vi "ClimberSetpointControl.vi"(11 "Buttons":bool[](array[boolean])) -> ()   [LabVIEW 2015]
uses:
  <vilib>/Rock Robotics/WPI/CAN/TalonSRX/WPI_CANTalonSRX_APIControlMode.ctl
  Utilities/MotorPositionGlobals.vi
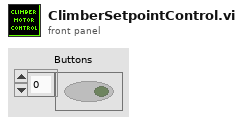
[diagram p1: front panel]
types:
  T1 = typedef "WPI_ServoDeviceRef.ctl" = cluster{"DeviceStatus":errorcluster, "PWM Channel":T2, "DeadBand":T3}
  T2 = typedef "FPGA_DIOPWMChannel.ctl" = enum8{"PWM 0", "PWM 1", "PWM 2", "PWM 3", "PWM 4", "PWM 5", "PWM 6", "PWM 7", "PWM 8", "PWM 9", "PWM MXP 0", "PWM MXP 1", "PWM MXP 2", "PWM MXP 3", "PWM MXP 4", "PWM MXP 5", "PWM MXP 6", "PWM MXP 7", "PWM MXP 8", "PWM MXP 9", "Invalid"}
  T3 = typedef "WPI_PWMDeadband.ctl" = cluster{"Name":string, "maxPositivePwm":i32, "minPositivePwm":i32, "centerPwm":i32, "maxNegativePwm":i32, "minNegativePwm":i32, "angularRange":u16}
  T4 = typedef "WPI_CANTalonSRX_APIControlMode.ctl" = enum8{"Percent VBus", "Speed", "Position", "Slave", "Unchanged / Invalid", "Voltage Compensation", "Current", "Motion Profile"}
  T5 = typedef "WPI_MotorControlDeviceRef.ctl" = cluster{"DeviceStatus":errorcluster, "Type":T6, "PWM":cluster{"PWM Channel":T2, "DeadBand":T3}, "CAN":cluster{"Device Number":u8, "Control Mode":T7, "Semaphore":T8, "Max Vout":dbl, "TalonSRX Control Mode":T4}, "Invert":bool}
  T6 = typedef "WPI_MotorControlType.ctl" = enum16{"PWM", "CAN", "CANTalonSRX"}
  T7 = typedef "WPI_CANJaguar_ControlMode.ctl" = enum8{"Percent VBus", "Current", "Speed", "Position", "Voltage"}
  T8 = typedef "Semaphore RefNum" = refnum<k1>
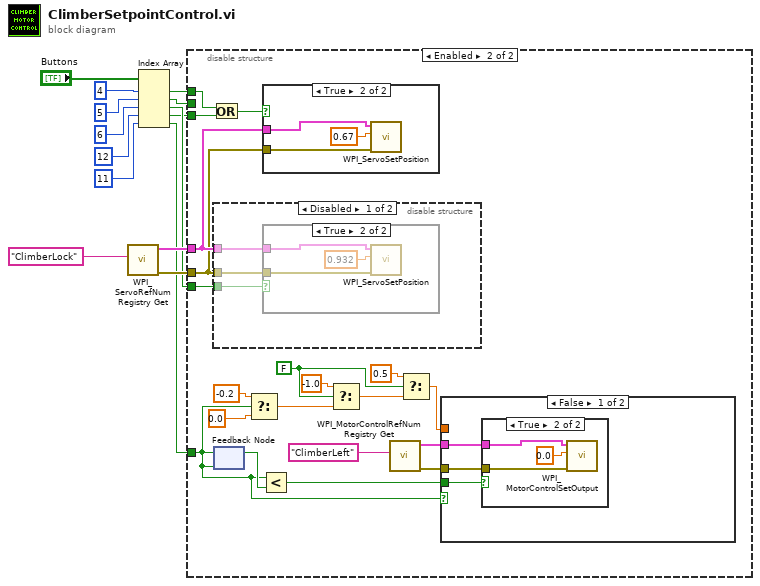
[diagram p0: block diagram]
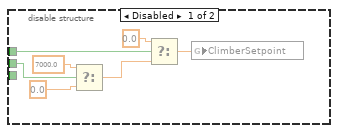
[diagram p2: hidden frame]
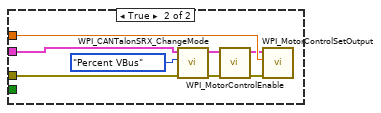
[diagram p4: hidden frame]
diagram:
  n1 = call <vilib>:"WPI_ServoRefNum Registry Get.vi"("refnum name"="ClimberLock") -> ("error out"=w6:errorcluster, "ServoDeviceRef"=w7:T1)  [unwired: 9 in]
  n2 = Index Array(array="Buttons", index #1=4 ("index"), index #2=5 ("index"), index #3=6 ("index"), index #4=12 ("index"), index #5=11 ("index")) -> (element #1=w11:bool, element #2=w10:bool, element #3=w5:bool, element #4=w3:bool, element #5=w1:bool)
  n3 = disable-structure shown="Enabled" {
    disable-tunnel: w11 -> [w17 w28]
    disable-tunnel: w10 -> [w16 _]
    disable-tunnel: w7 -> [_ w33]
    disable-tunnel: w6 -> [_ w32]
    disable-tunnel: w5 -> [_ w35]
    disable-tunnel: w3 -> [_ w34]
    disable-tunnel: w1 -> [_ w23]
    frame Disabled {
      n4 = Select(t=7000.0, s=w16, f=0.0) -> (s? t:f=w20:dbl)
      n5 = Select(t=0.0, s=w17, f=w20) -> (s? t:f=w15:dbl)
      n6 = global write "MotorPositionGlobals.vi" "ClimberSetpoint"(w15) -> ()
    }
    frame Enabled {
      w26 = FALSE ("s")
      n7 = Or(x=w28, y=w34) -> (x .or. y?=w27:bool)
      n8 = disable-structure shown="Disabled" {
        disable-tunnel: w35 -> [w58 _]
        disable-tunnel: w33 -> [w57 _]
        disable-tunnel: w32 -> [w56 _]
        frame Disabled {
          n9 = case shown="True" w58 {
            tunnel: w57 -> [_ w61]
            tunnel: w56 -> [_ w60]
            frame False {
            }
            frame True {
              n10 = call <vilib>:"WPI_ServoSetPosition.vi"("error in (no error)"=w60, "Position"=0.932, "ServoDeviceRef"=w61) -> ()  [unwired: 7 in, 2 out]
            }
          }
        }
        frame Enabled {
        }
      }
      n11 = feedback-in #1(w23) -> ()
      n12 = feedback #1(w23) -> (w24:bool)
      n13 = Select(t=-0.2, s=w23, f=0.0) -> (s? t:f=w30:dbl)
      n14 = Less?(x=w23, y=w24) -> (x < y?=w22:bool)
      n15 = case shown="True" w27 {
        tunnel: w33 -> [_ w63]
        tunnel: w32 -> [_ w62]
        frame False {
        }
        frame True {
          n16 = call <vilib>:"WPI_ServoSetPosition.vi"("error in (no error)"=w62, "Position"=0.67, "ServoDeviceRef"=w63) -> ()  [unwired: 7 in, 2 out]
        }
      }
      n17 = Select(t=-1.0, s=w26, f=w30) -> (s? t:f=w38:dbl)
      n18 = call <vilib>:"WPI_MotorControlRefNum Registry Get.vi"("refnum name"="ClimberLeft") -> ("error out"=w39:errorcluster, "MotorControlDevRef"=w25:T5)  [unwired: 9 in]
      n19 = Select(t=0.5, s=w26, f=w38) -> (s? t:f=w36:dbl)
      n20 = case shown="False" w23 {
        tunnel: w39 -> [w42 w54]
        tunnel: w36 -> [_ w55]
        tunnel: w25 -> [w43 w53]
        tunnel: w22 -> [w44 _]
        frame False {
          n21 = case shown="True" w44 {
            tunnel: w43 -> [_ w47]
            tunnel: w42 -> [_ w46]
            frame False {
            }
            frame True {
              n22 = call <vilib>:"WPI_MotorControlSetOutput.vi"("error in (no error)"=w46, "Output"=0.0, "MotorControlDevRef"=w47) -> ()  [unwired: 6 in, 3 out]
            }
          }
        }
        frame True {
          n23 = call <vilib>:"WPI_CANTalonSRX_ChangeMode.vi"("error in (no error)"=w54, "Control Mode"=WPI_CANTalonSRX_APIControlMode."Percent VBus", "CAN Talon SRX Ref"=w53) -> ("error out"=w51:errorcluster, "CAN Talon SRX Ref"=w50:T5)  [unwired: 7 in]
          n24 = call <vilib>:"WPI_MotorControlEnable.vi"("error in (no error)"=w51, "CAN MotorDevRef"=w50) -> ("error out"=w48:errorcluster, "CAN MotorDevRef"=w49:T5)  [unwired: 8 in]
          n25 = call <vilib>:"WPI_MotorControlSetOutput.vi"("error in (no error)"=w48, "Output"=w55, "MotorControlDevRef"=w49) -> ()  [unwired: 6 in, 3 out]
        }
      }
    }
  }
